vi "lasercall.vi"   [LabVIEW 2013]
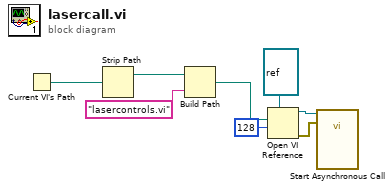
[diagram p0: block diagram]
diagram:
  n1 = Current VI's Path() -> (path=w4:path)
  n2 = Strip Path(path=w4) -> (stripped path=w5:path)  [unwired: 1 out]
  n3 = Build Path(base path=w5, name or relative path="lasercontrols.vi") -> (appended path=w3:path)
  n4 = Open VI Reference(type specifier VI Refnum (for type only)=refnum<vi> refnum, vi path=w3, options=128) -> (vi reference=w7:refnum<vi>, error out=w8:errorcluster)  [unwired: 3 in]
  n5 = call-by-ref "Start Asynchronous Call"(reference=w7, error in=w8) -> ()  [unwired: 1 in, 2 out]
